vi "Pixel Value (-1 to 1) AE.vi"(2 "Action":T1, 7 "Pixel Value (-1 to 1)":dbl[](array[numeric])) -> (8 "Pixel Value (-1 to 1) Out":dbl[](array[numeric]))   [LabVIEW 2014]
uses:
  Standard Action.ctl
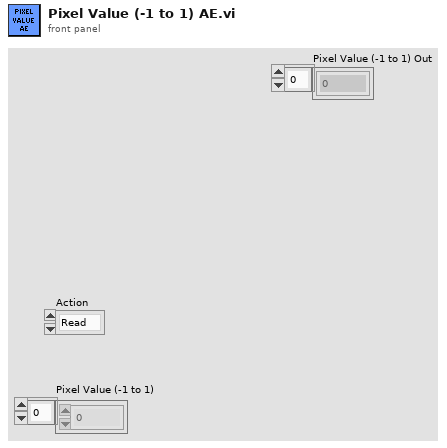
[diagram p1: front panel]
types:
  T1 = typedef "Standard Action.ctl" = enum16{"Read", "Write"}
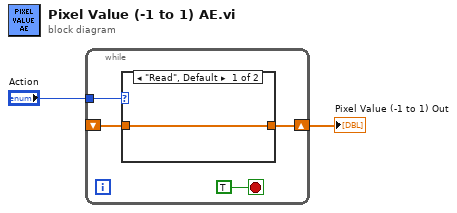
[diagram p0: block diagram]
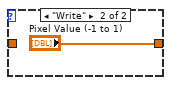
[diagram p2: hidden frame]
diagram:
  n1 = while {
    shift-right: [w4] -> w1
    shift-left: _ -> [w3]
    tunnel: "Action" -> [w5]
    stop <- TRUE stop-if-true
    n2 = case shown="\"Read\", Default" w5 {
      tunnel: [w7 "Pixel Value (-1 to 1)"] -> w4
      tunnel: w3 -> [w7 _]
      frame "Read", Default {
      }
      frame "Write" {
      }
    }
  }
  "Pixel Value (-1 to 1) Out" <- w1
